vi "Replace Aliases with Endpoints.vi"(10 "Alias Mappings":T2[](array[typedef]), 11 "UI Connections List in":T1[](array[typedef])) -> (3 "UI Connections List out":T1[](array[typedef]))   [LabVIEW 2017, in "Routing and Faulting System Explorer.lvlib"]
uses:
  Routing and Faulting System Explorer.lvlib
  Shared/Alias Mapping.ctl
  Connection Row.ctl
  Shared/Routing and Faulting Shared.lvlib
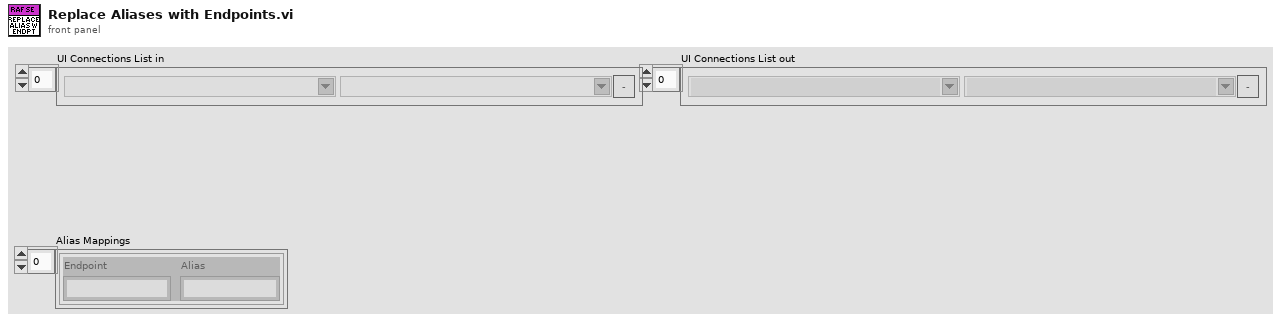
[diagram p1: front panel]
types:
  T1 = typedef "Routing and Faulting System Explorer.lvlib/Connection Row.ctl" = cluster{"Source":string, "Destination":string, "Remove":bool}
  T2 = typedef "Routing and Faulting Shared.lvlib/Alias Mapping.ctl" = cluster{"Endpoint":string, "Alias":string}
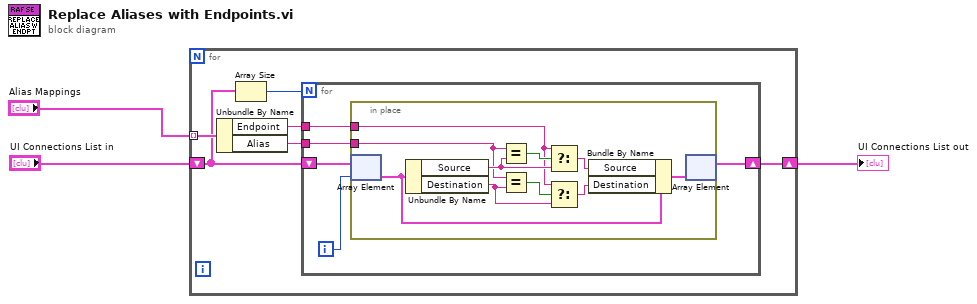
[diagram p0: block diagram]
diagram:
  n1 = for {
    tunnel: "Alias Mappings" -> [w9] mode=indexing
    shift-right: [w6] -> w2
    shift-left: "UI Connections List in" -> [w5]
    n2 = Unbundle By Name(w9) -> ("Endpoint"=w8:string, "Alias"=w7:string)
    n3 = Array Size(array=w5) -> (size(s)=w4:i32)
    n4 = for {
      N: w4 -> [_]
      tunnel: w8 -> [w13]
      tunnel: w7 -> [w12]
      shift-right: [w11] -> w6
      shift-left: w5 -> [w14]
      i -> [w10]
      n5 = in-place {
        in-place-border: w13 -> [w16]
        in-place-border: w12 -> [w15]
        n6 = in-place-array #1(w14, w10) -> (w18:T1)
        n7 = Unbundle By Name(w18) -> ("Source"=w21:string, "Destination"=w23:string)
        n8 = Equal?(x=w15, y=w21) -> (x = y?=w19:bool)
        n9 = Equal?(x=w15, y=w23) -> (x = y?=w22:bool)
        n10 = Select(t=w16, s=w19, f=w21) -> (s? t:f=w20:string)
        n11 = Select(t=w16, s=w22, f=w23) -> (s? t:f=w24:string)
        n12 = Bundle By Name(cluster=w18, "Source"=w20, "Destination"=w24) -> (w17:T1)
        n13 = in-place-array #1(w17) -> (w11:T1[])  [unwired: 1 out]
      }
    }
  }
  "UI Connections List out" <- w2
